vi "Serial_Escape.vi"(4 "data":u8[](array[numeric]) format="%.0x") -> (1 "data out":u8[](array[numeric]) format="%.0x")   [LabVIEW 2009, in "Serial.lvlib"]
doc: "Escapes the following bytes in the data:\n0xFF byte in data is replaced by sequence 0xFE 0xFE\n0xFE byte in data is replaced by 0xFE 0xFD sequence"
uses:
  Serial.lvlib
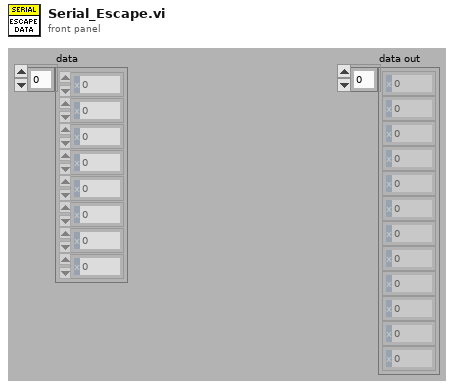
[diagram p1: front panel]
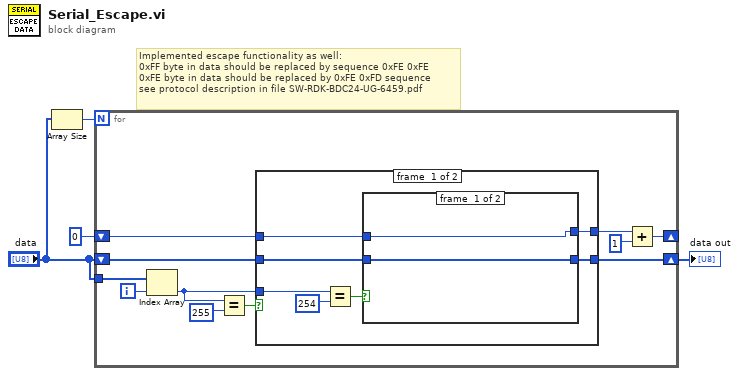
[diagram p0: block diagram]
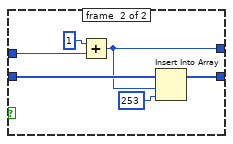
[diagram p2: hidden frame]
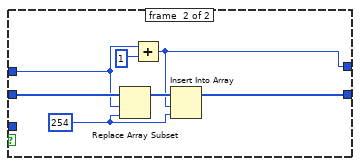
[diagram p3: hidden frame]
diagram:
  # "Implemented escape functionality as well:\n0xFF byte in data should be replaced by sequence 0xFE 0xFE\n0xFE byte in data should be replaced by 0xFE 0xFD sequence\nsee protocol description in file SW-RDK-BDC24-UG-6459.pdf"
  n1 = Array Size(array="data") -> (size(s)=w3:i32)
  n2 = for {
    N: w3 -> [_]
    tunnel: "data" -> [w12]
    shift-right: [w13] -> w4
    shift-left: "data" -> [w9]
    shift-right: [w6] -> _
    shift-left: 0 ("Numeric") -> [w5]
    i -> [w10]
    n3 = Index Array(array=w12, index=w10) -> (element=w11:u8)
    n4 = Equal?(x=w11, y=u8 255 ("element")) -> (x = y?=w14:bool)
    n5 = case shown="False" w14 {
      tunnel: w9 -> [w19 w37]
      tunnel: [w18 w32] -> w13
      tunnel: w11 -> [w21 _]
      tunnel: w5 -> [w17 w35]
      tunnel: [w16 w31] -> w8
      frame #0 {
        n6 = Equal?(x=w21, y=u8 254) -> (x = y?=w22:bool)
        n7 = case shown="True" w22 {
          tunnel: w19 -> [w24 w30]
          tunnel: [w24 w26] -> w18
          tunnel: w17 -> [w23 w29]
          tunnel: [w23 w25] -> w16
          frame #0 {
          }
          frame #1 {
            n8 = Add(x=1, y=w29) -> (x+y=w25:i32)
            n9 = Insert Into Array(array=w30, index=w25, new element=u8 253 ("new element/subarray")) -> (w26:u8[])
          }
        }
      }
      frame #1 {
        w33 = u8 254 ("new element/subarray")
        n10 = Replace Array Subset(array=w37, new element=w33, index=w35) -> (w36:u8[])
        n11 = Add(x=w35, y=1) -> (x+y=w31:i32)
        n12 = Insert Into Array(array=w36, index=w31, new element=w33) -> (w32:u8[])
      }
    }
    n13 = Add(x=w8, y=1) -> (x+y=w6:i32)
  }
  "data out" <- w4
